vi "Compile Routing and Faulting Configuration.vi"(6 "Get Channel Data Refnum":refnum<vi>, 8 "error in (no error)":errorcluster, 10 "Communication Configuration":T1, 11 "Device Ref in":T2 format="%.0x") -> (0 "error out":errorcluster, 2 "RaF Configuration":T3, 3 "Device Ref out":T2 format="%.0x")   [LabVIEW 2020, in "Routing and Faulting System Explorer.lvlib"]
uses:
  Routing and Faulting System Explorer.lvlib
  Shared/Routing and Faulting Configuration.ctl
  Shared/Routing Channel Configuration.ctl
  Shared/Value-Connections Map.ctl
  Shared/Alias Mapping.ctl
  Shared/Alias Endpoint.ctl
  Shared/Compiled Connection.ctl
  <vilib>/NI VeriStand/Custom Device API/Custom Device Item Ref.ctl
  Shared/Communication Configuration.ctl
  Shared/Routing and Faulting Shared.lvlib
  <vilib>/NI VeriStand/Custom Device API/Custom Device API.lvlib
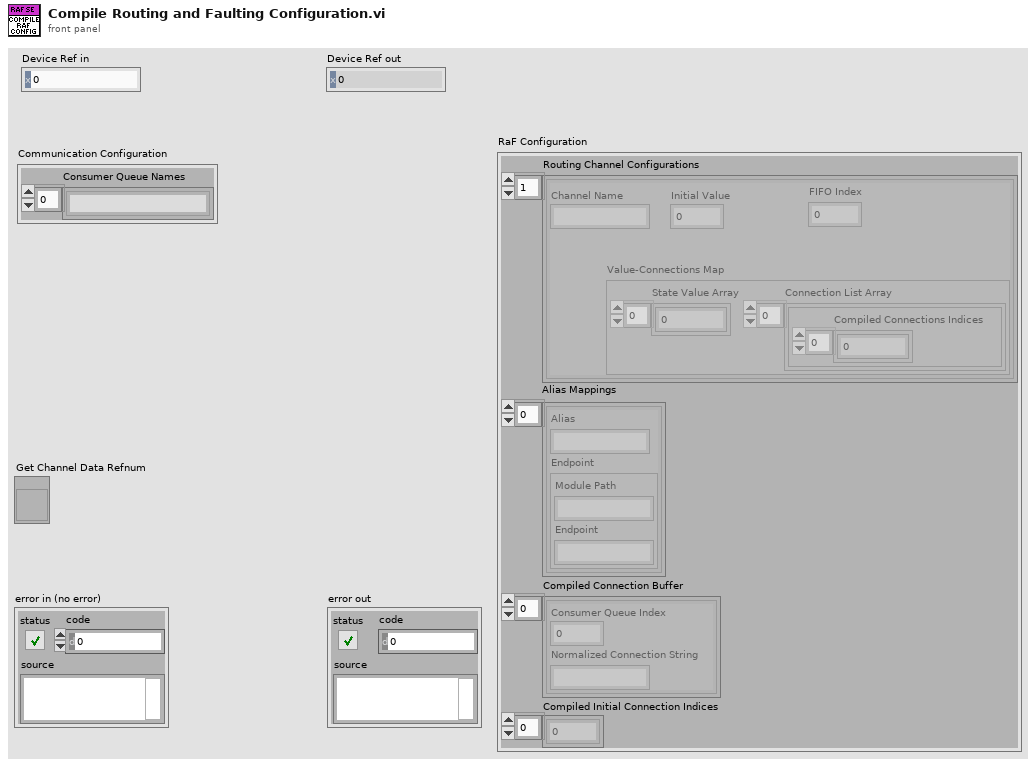
[diagram p1: front panel]
types:
  T1 = typedef "Routing and Faulting Shared.lvlib/Communication Configuration.ctl" = cluster{"Consumer Queue Names":string[]}
  T2 = typedef "Custom Device API.lvlib/Custom Device Item Ref.ctl" = u64
  T3 = typedef "Routing and Faulting Shared.lvlib/Routing and Faulting Configuration.ctl" = cluster{"Routing Channel Configurations":T4[], "Alias Mappings":T6[], "Compiled Connection Buffer":T8[], "Compiled Initial Connection Indices":i32[]}
  T4 = typedef "Routing and Faulting Shared.lvlib/Routing Channel Configuration.ctl" = cluster{"Channel Name":string, "Initial Value":dbl, "FIFO Index":i32, "Value-Connections Map":T5}
  T5 = typedef "Routing and Faulting Shared.lvlib/Value-Connections Map.ctl" = cluster{"State Value Array":i32[], "Connection List Array":cluster{"Compiled Connections Indices":i32[]}[]}
  T6 = typedef "Routing and Faulting Shared.lvlib/Alias Mapping.ctl" = cluster{"Alias":string, "Endpoint":T7}
  T7 = typedef "Routing and Faulting Shared.lvlib/Alias Endpoint.ctl" = cluster{"Module Path":string, "Endpoint":string}
  T8 = typedef "Routing and Faulting Shared.lvlib/Compiled Connection.ctl" = cluster{"Consumer Queue Index":i32, "Normalized Connection String":string}
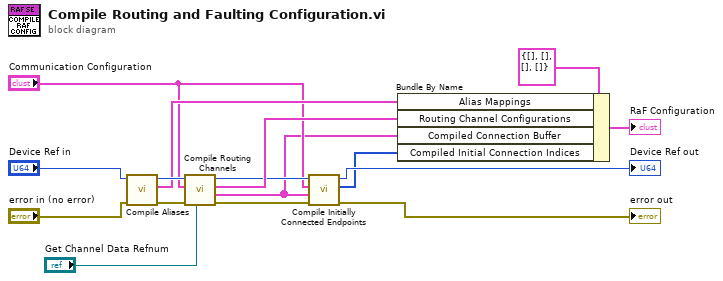
[diagram p0: block diagram]
diagram:
  n1 = call "Compile Aliases.vi"("error in (no error)"="error in (no error)", "Device Ref in"="Device Ref in") -> ("error out"=w11:errorcluster, "Alias Mappings"=w10:T6[], "Device Ref out"=w12:T2)  [unwired: 7 in]
  n2 = call "Compile Routing Channels.vi"("Get Channel Data Refnum"="Get Channel Data Refnum", "error in (no error)"=w11, "Communication Configuration"="Communication Configuration", "Device Ref in"=w12) -> ("error out"=w7:errorcluster, "Compiled Connections Buffer"=w2:T8[], "Routing Channels Configuration"=w8:T4[], "Device Ref out"=w5:T2)  [unwired: 4 in]
  n3 = call "Compile Initially Connected Endpoints.vi"("error in"=w7, "Compiled Connections Buffer"=w2, "Communication Configuration"="Communication Configuration", "Device Ref in"=w5) -> ("error out"=→"error out":errorcluster, "Compiled Initial Connection Indices"=w1:i32[], "Device Ref out"=→"Device Ref out":T2)  [unwired: 5 in]
  n4 = Bundle By Name(cluster=T3 {"Routing Channel Configurations"=[], "Alias Mappings"=[], "Compiled Connection Buffer"=[], "Compiled Initial Connection Indices"=[]} ("Routing and Faulting Configuration"), "Alias Mappings"=w10, "Routing Channel Configurations"=w8, "Compiled Connection Buffer"=w2, "Compiled Initial Connection Indices"=w1) -> (→"RaF Configuration":T3)
